vi "test2-ErrorStr conversion.vi"(8 "error in (no error)":errorcluster, 11 "TestCase in":refnum<class "testcase-CSMArgument.lvclass">) -> (0 "error out":errorcluster, 3 "TestCase out":refnum<class "testcase-CSMArgument.lvclass">)   [LabVIEW 2017, in "testcase-CSMArgument.lvclass"]
uses:
  testcase-CSMArgument.lvclass
  src/user.lib/_NEVSTOP/Communicable State Machine(CSM)/AdvanceAPI/CSM - Revert Arguments-Safe String.vi
  src/user.lib/_NEVSTOP/Communicable State Machine(CSM)/AdvanceAPI/CSM - Make String Arguments Safe.vi
  src/user.lib/_NEVSTOP/Communicable State Machine(CSM)/AdvanceAPI/CSM - Keywords.vi
  src/user.lib/_NEVSTOP/Communicable State Machine(CSM)/_Shared/Trim Single-line Text.vi
  <vilib>/addons/_JKI Toolkits/VI Tester/TestCase.llb/TestCase.lvclass
  src/user.lib/_NEVSTOP/Communicable State Machine(CSM)/Communicable State Machine.lvlib
  src/user.lib/_NEVSTOP/Communicable State Machine(CSM)/_Shared/CSM Shared.lvlib
  C:/Program Files (x86)/National Instruments/LabVIEW 2017/vi.lib/addons/_JKI Toolkits/VI Tester/TestCase.llb/TestCase.lvclass
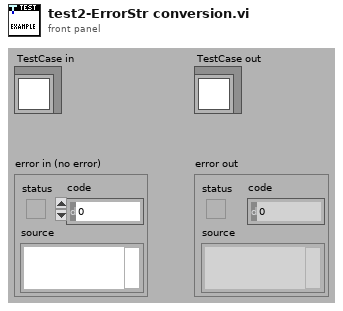
[diagram p1: front panel]
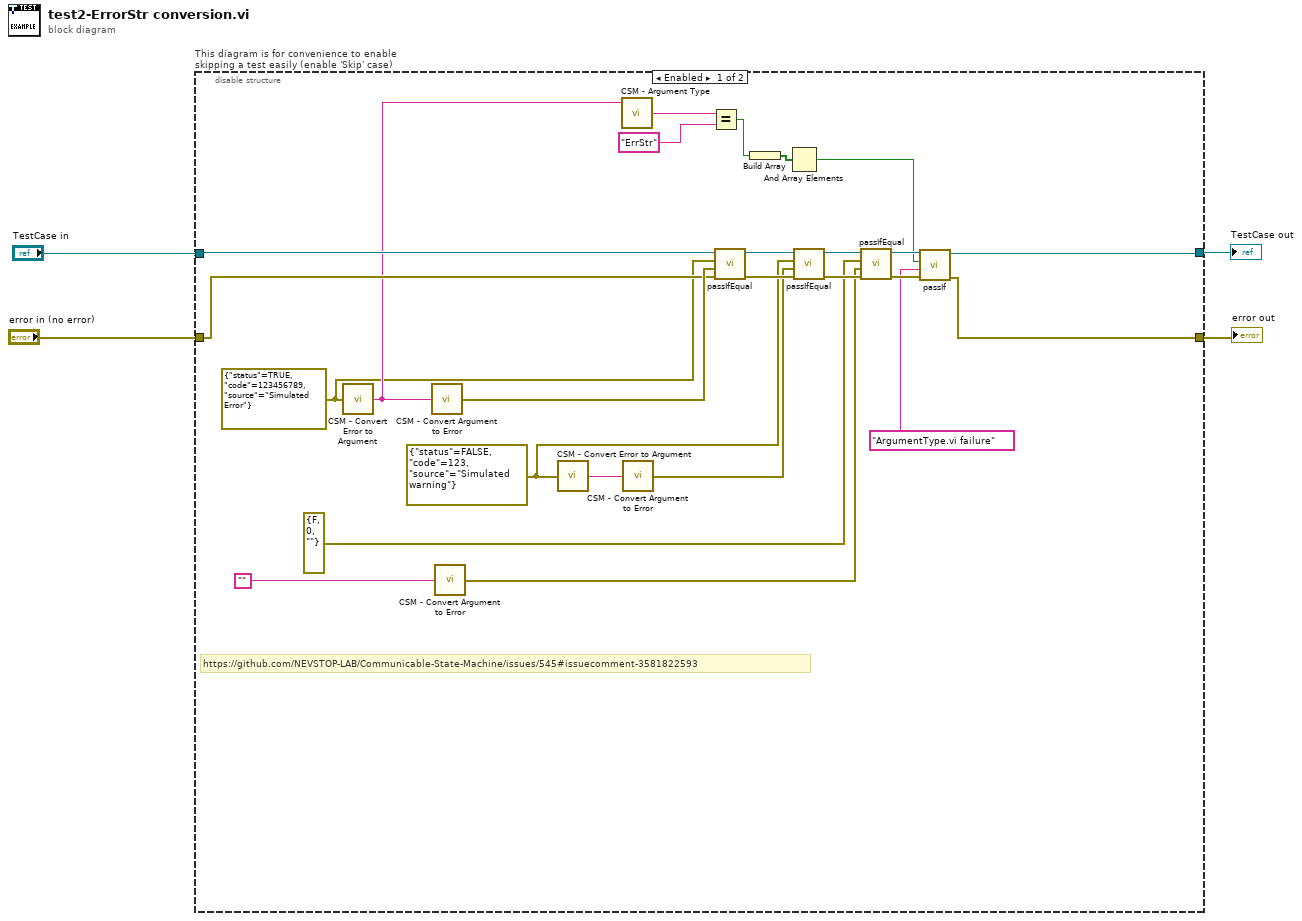
[diagram p0: block diagram]
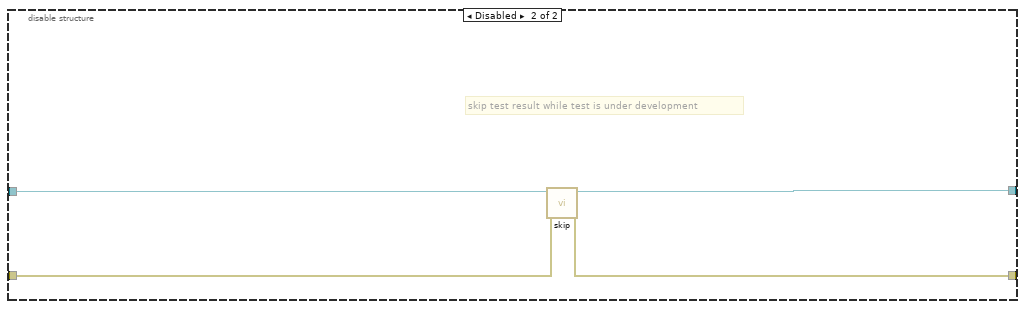
[diagram p2: hidden frame]
diagram:
  n1 = disable-structure "This diagram is for convenience to enable skipping a test easily (enable 'Skip' case)" shown="Enabled" {
    disable-tunnel: "TestCase in" -> [w29 w33]
    disable-tunnel: [w11 w31] -> w1
    disable-tunnel: [w13 w32] -> w3
    disable-tunnel: "error in (no error)" -> [w23 w30]
    frame Enabled {
      w7 = errorcluster {"status"=FALSE, "code"=123, "source"="Simulated warning"} ("error constant")
      w5 = errorcluster {"status"=TRUE, "code"=123456789, "source"="Simulated Error"} ("error constant")
      # "https://github.com/NEVSTOP-LAB/Communicable-State-Machine/issues/545#issuecomment-3581822593"
      n2 = call "CSM - Convert Error to Argument.vi"("Error"=w5) -> ("Argument"=w16:string)  [unwired: 4 in]
      n3 = call "CSM - Convert Argument to Error.vi"("Argument"=w16) -> ("Error"=w24:errorcluster)  [unwired: 4 in]
      n4 = call "CSM - Convert Argument to Error.vi"("Argument"="") -> ("Error"=w20:errorcluster)  [unwired: 4 in]
      n5 = call "CSM - Convert Error to Argument.vi"("Error"=w7) -> ("Argument"=w15:string)  [unwired: 4 in]
      n6 = call "CSM - Argument Type.vi"("Arguments"=w16) -> ("Argument Type"=w17:string)  [unwired: 3 in, 1 out]
      n7 = call "CSM - Convert Argument to Error.vi"("Argument"=w15) -> ("Error"=w22:errorcluster)  [unwired: 4 in]
      n8 = Equal?(x=w17, y="ErrStr") -> (x = y?=w19:bool)
      n9 = call-dynamic "passIfEqual.vi"("error in (no error)"=w23, "y"=w24, "x"=w5, "TestCase in"=w29) -> ("error out"=w27:errorcluster, "TestCase out"=w28:refnum<class "testcase-CSMArgument.lvclass">)  [unwired: 6 in]
      n10 = Build Array(w19) -> (w18:bool[])
      n11 = And Array Elements(Boolean array=w18) -> (logical AND=w10:bool)
      n12 = call-dynamic "passIfEqual.vi"("error in (no error)"=w27, "y"=w22, "x"=w7, "TestCase in"=w28) -> ("error out"=w25:errorcluster, "TestCase out"=w26:refnum<class "testcase-CSMArgument.lvclass">)  [unwired: 6 in]
      n13 = call-dynamic "passIfEqual.vi"("error in (no error)"=w25, "y"=w20, "x"=errorcluster {"status"=FALSE, "code"=0, "source"=""} ("error constant"), "TestCase in"=w26) -> ("error out"=w14:errorcluster, "TestCase out"=w12:refnum<class "testcase-CSMArgument.lvclass">)  [unwired: 6 in]
      n14 = call-dynamic "passIf.vi"("error in (no error)"=w14, "message (\"\")"="ArgumentType.vi failure" ("message (\"\")"), "pass"=w10, "TestCase in"=w12) -> ("error out"=w13:errorcluster, "TestCase out"=w11:refnum<class "testcase-CSMArgument.lvclass">)  [unwired: 6 in]
    }
    frame Disabled {
      # "skip test result while test is under development"
      n15 = call <vilib>:"skip.vi"("error in (no error)"=w30, "TestCase in"=w33) -> ("error out"=w32:errorcluster, "TestCase out"=w31:refnum<class "testcase-CSMArgument.lvclass">)  [unwired: 8 in]
    }
  }
  "error out" <- w3
  "TestCase out" <- w1
